vi "ReadCursor_pos.vi"(8 "error in (no error)":errorcluster, 11 "object in":refnum<class "inspect_request Message.lvclass">) -> (0 "error out":errorcluster, 2 "cursor_pos":u32, 3 "object out":refnum<class "inspect_request Message.lvclass">)   [LabVIEW 2018, in "ClientMessaging.lvlib" / "inspect_request Message.lvclass"]
uses:
  inspect_request Message.lvclass
  inspect_request Message.lvclass/inspect_request Message.ctl
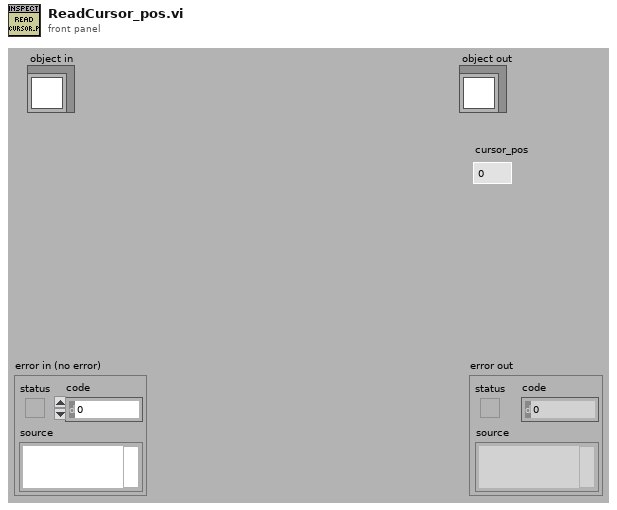
[diagram p1: front panel]
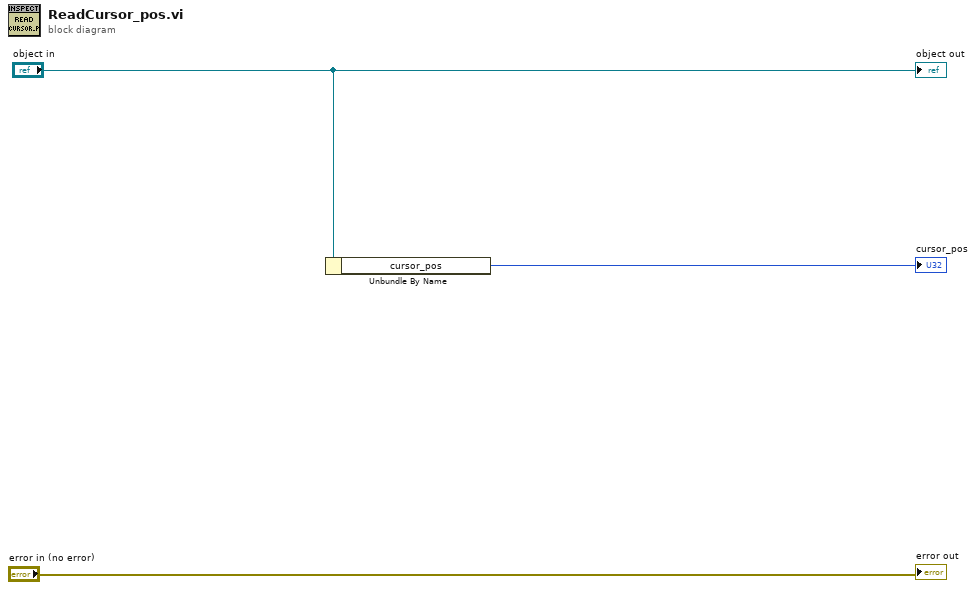
[diagram p0: block diagram]
diagram:
  n1 = Unbundle By Name("object in") -> ("cursor_pos"=→"cursor_pos":u32)
  "error out" <- "error in (no error)"
  "object out" <- "object in"
